vi "DriveModuleControl.vi"(8 "error in":errorcluster, 9 "Actual State":T1={"Speed"=0.0, "Angle"={"VALUE"=0.0, "COS"=1.0, "SIN"=0.0}} {"Angle"."SIN" format="%13.4f"; "Angle"."COS" format="%13.4f"; "Angle"."VALUE" format="%13.4f"}, 10 "Desired State":T1={"Speed"=0.0, "Angle"={"VALUE"=0.0, "COS"=1.0, "SIN"=0.0}} {"Angle"."SIN" format="%13.4f"; "Angle"."COS" format="%13.4f"; "Angle"."VALUE" format="%13.4f"}, 11 "ModualNamePrefix":i32) -> (0 "error out":errorcluster)   [LabVIEW 2023]
uses:
  <vilib>/Rock Robotics/WPI/ThirdParty/JAS_Junk/TrajLib/TypeDef/SWERVE_DRIVE_MODULE_STATE.ctl
  <vilib>/Rock Robotics/WPI/ThirdParty/JAS_Junk/TrajLib/TypeDef/ROTATION2D.ctl
  <vilib>/Rock Robotics/WPI/ThirdParty/JAS_Junk/TrajLib/Rotation2d_Minus.vi
  <vilib>/Rock Robotics/WPI/ThirdParty/JAS_Junk/TrajLib/Rotation2d_GetRadians.vi
  <vilib>/Rock Robotics/WPI/ThirdParty/JAS_Junk/TrajLib/SwerveModuleState_New.vi
  <vilib>/Rock Robotics/WPI/ThirdParty/JAS_Junk/TrajLib/Rotation2d_RotateBy.vi
  <vilib>/Rock Robotics/WPI/ThirdParty/JAS_Junk/TrajLib/Rotation2d_CreateAngle.vi
  <vilib>/Rock Robotics/WPI/ThirdParty/JAS_Junk/TrajLib/SimpleMotorFF_Calculate.vi
  <vilib>/Rock Robotics/WPI/ThirdParty/JAS_Junk/TrajLib/PIDController_AtSetpoint.vi
  <vilib>/Rock Robotics/WPI/ThirdParty/JAS_Junk/TrajLib/PIDController_SetPIDF.vi
  <vilib>/Rock Robotics/WPI/ThirdParty/JAS_Junk/TrajLib/PIDController_SetDerivativeFilter.vi
  <vilib>/Rock Robotics/WPI/ThirdParty/JAS_Junk/TrajLib/PIDController_SetIntegratorRange.vi
  <vilib>/Rock Robotics/WPI/ThirdParty/JAS_Junk/TrajLib/PIDController_SetTolerancePandV.vi
  <vilib>/Rock Robotics/WPI/ThirdParty/JAS_Junk/TrajLib/PIDController_DisableContinousInput.vi
  <vilib>/Rock Robotics/WPI/ThirdParty/JAS_Junk/TrajLib/PIDController_EnableContinousInput.vi
  <vilib>/Rock Robotics/WPI/ThirdParty/JAS_Junk/TrajLib/PIDController_Reset.vi
  <vilib>/Rock Robotics/WPI/ThirdParty/JAS_Junk/TrajLib/PIDController_New.vi
  <vilib>/Rock Robotics/WPI/ThirdParty/JAS_Junk/TrajLib/PIDController_SetOutputLimits.vi
  <vilib>/Rock Robotics/WPI/ThirdParty/JAS_Junk/TrajLib/VI/PIDController_SetIntegratorZone.vi
  <vilib>/Rock Robotics/WPI/ThirdParty/JAS_Junk/TrajLib/SlewRateLimiter_New.vi
  <vilib>/Rock Robotics/WPI/ThirdParty/JAS_Junk/TrajLib/SlewRateLimiter_Reset.vi
  <vilib>/Rock Robotics/WPI/ThirdParty/JAS_Junk/TrajLib/SlewRateLimiter_Calculate.vi
  <vilib>/Rock Robotics/WPI/ThirdParty/JAS_Junk/TrajLib/SlewRateLimiter_SetRate.vi
  <vilib>/Rock Robotics/WPI/ThirdParty/JAS_Junk/TrajLib/Rotation2d_UnaryMinus.vi
  <vilib>/Rock Robotics/WPI/ThirdParty/JAS_Junk/TrajLib/Rotation2d_CreateXY.vi
  <vilib>/Rock Robotics/WPI/ThirdParty/JAS_Junk/TrajLib/PIDController_NewPeriod.vi
  <vilib>/Rock Robotics/WPI/ThirdParty/JAS_Junk/TrajLib/Util_GetTime.vi
  <vilib>/Rock Robotics/WPI/ThirdParty/JAS_Junk/TrajLib/Util_CalcDist.vi
  <vilib>/Rock Robotics/SystemInterfaces/NetworkCommunication/NetComm_UsageReport_report.vi
  <vilib>/Rock Robotics/WPI/ThirdParty/JAS_Junk/TrajLib/VI/Util_GetTime_U32.vi
  DriveGlobal.vi
  <vilib>/Rock Robotics/SystemInterfaces/Utilities/FPGA_UtilitiesRead LocalTime.vi
  <vilib>/Rock Robotics/WPI/ThirdParty/JAS_Junk/TrajLib/VI/Util_GetTime_U64.vi
  <vilib>/Rock Robotics/WPI/ThirdParty/Phoenix6/Phoenix6_Device_RefNumRegistryGet.vi
  <vilib>/Rock Robotics/WPI/MotorControl/WPI_MotorControlRefNum Registry Get.vi
  <vilib>/Rock Robotics/WPI/ThirdParty/JAS_Junk/TrajLib/Globals/Util_LibraryGlobals.vi
  <vilib>/Rock Robotics/WPI/ThirdParty/JAS_Junk/TrajLib/PIDController_AdvCalculate_FF_Sp_Pv.vi
  <vilib>/Rock Robotics/WPI/ThirdParty/JAS_Junk/TrajLib/Trajectory_Library.lvlib
  <vilib>/Rock Robotics/Network Tables/NT Write Number.vi
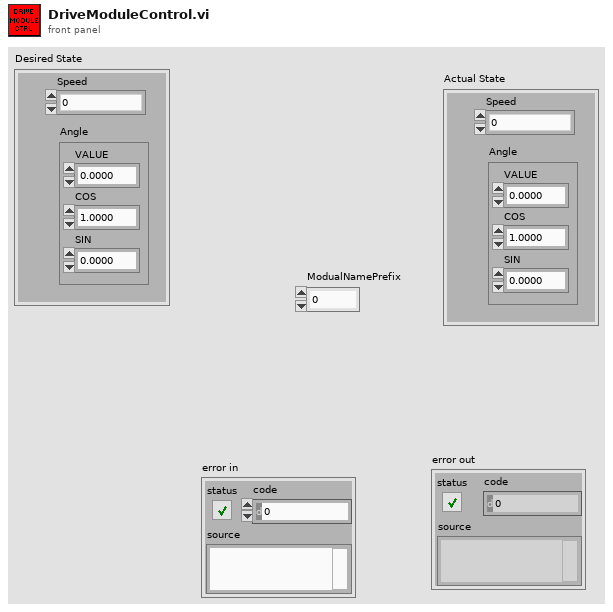
[diagram p1: front panel]
types:
  T1 = typedef "Trajectory_Library.lvlib/SWERVE_DRIVE_MODULE_STATE.ctl" = cluster{"Speed":dbl, "Angle":T2}
  T2 = typedef "Trajectory_Library.lvlib/ROTATION2D.ctl" = cluster{"VALUE":dbl, "COS":dbl, "SIN":dbl}
  T3 = typedef "WPI_MotorControlDeviceRef.ctl" = cluster{"DeviceStatus":errorcluster, "Type":T4, "PWM":cluster{"PWM Channel":T5, "DeadBand":T6}, "CAN":cluster{"Device Number":u8, "SetOutput VI Ref":variant, "GetOutput VI Ref":variant, "Enable VI Ref":variant, "Disable VI Ref":variant, "Data":variant}, "Invert":bool, "DIO PWM":cluster{"PWM \"Enable\" Channel":T5, "DIOChannel":T7, "PWM Rate":dbl}}
  T4 = typedef "WPI_MotorControlType.ctl" = enum16{"PWM", "CAN", "DIO PWM"}
  T5 = typedef "FPGA_DIOPWMChannel.ctl" = enum8{"PWM 0", "PWM 1", "PWM 2", "PWM 3", "PWM 4", "PWM 5", "PWM 6", "PWM 7", "PWM 8", "PWM 9", "PWM MXP 0", "PWM MXP 1", "PWM MXP 2", "PWM MXP 3", "PWM MXP 4", "PWM MXP 5", "PWM MXP 6", "PWM MXP 7", "PWM MXP 8", "PWM MXP 9", "Invalid"}
  T6 = typedef "WPI_PWMDeadband.ctl" = cluster{"Name":string, "maxPositivePwm":i32, "minPositivePwm":i32, "centerPwm":i32, "maxNegativePwm":i32, "minNegativePwm":i32, "angularRange":u16}
  T7 = typedef "FPGA_DIOChannel.ctl" = enum8{"DIO 0", "DIO 1", "DIO 2", "DIO 3", "DIO 4", "DIO 5", "DIO 6", "DIO 7", "DIO 8", "DIO 9", "DIO MXP 0", "DIO MXP 1", "DIO MXP 2", "DIO MXP 3", "DIO MXP 4", "DIO MXP 5", "DIO MXP 6", "DIO MXP 7", "DIO MXP 8", "DIO MXP 9", "DIO MXP 10", "DIO MXP 11", "DIO MXP 12", "DIO MXP 13", "DIO MXP 14", "DIO MXP 15", "SPI Port CS1", "SPI Port CS2", "SPI Port CS3", "SPI Port MISO", "SPI Port MOSI", "Invalid"}
  T8 = typedef "Trajectory_Library.lvlib/SIMPLE_MOTOR_FF.ctl" = cluster{"Ks":dbl, "Kv":dbl, "Ka":dbl, "KnInv":dbl}
  T9 = typedef "Trajectory_Library.lvlib/PID_ADV_LIMITS.ctl" = cluster{"MaxInput":dbl, "MinInput":dbl, "Continuous":bool, "MaxOutput":dbl, "MinOutput":dbl}
  T10 = typedef "Trajectory_Library.lvlib/PID_ADV_TUNING.ctl" = cluster{"Kf":dbl, "Kp":dbl, "Ki":dbl, "Kd":dbl, "MaximumIntegral":dbl, "MinimumIntegral":dbl, "Filter Derivative":bool, "IntegralZone":dbl}
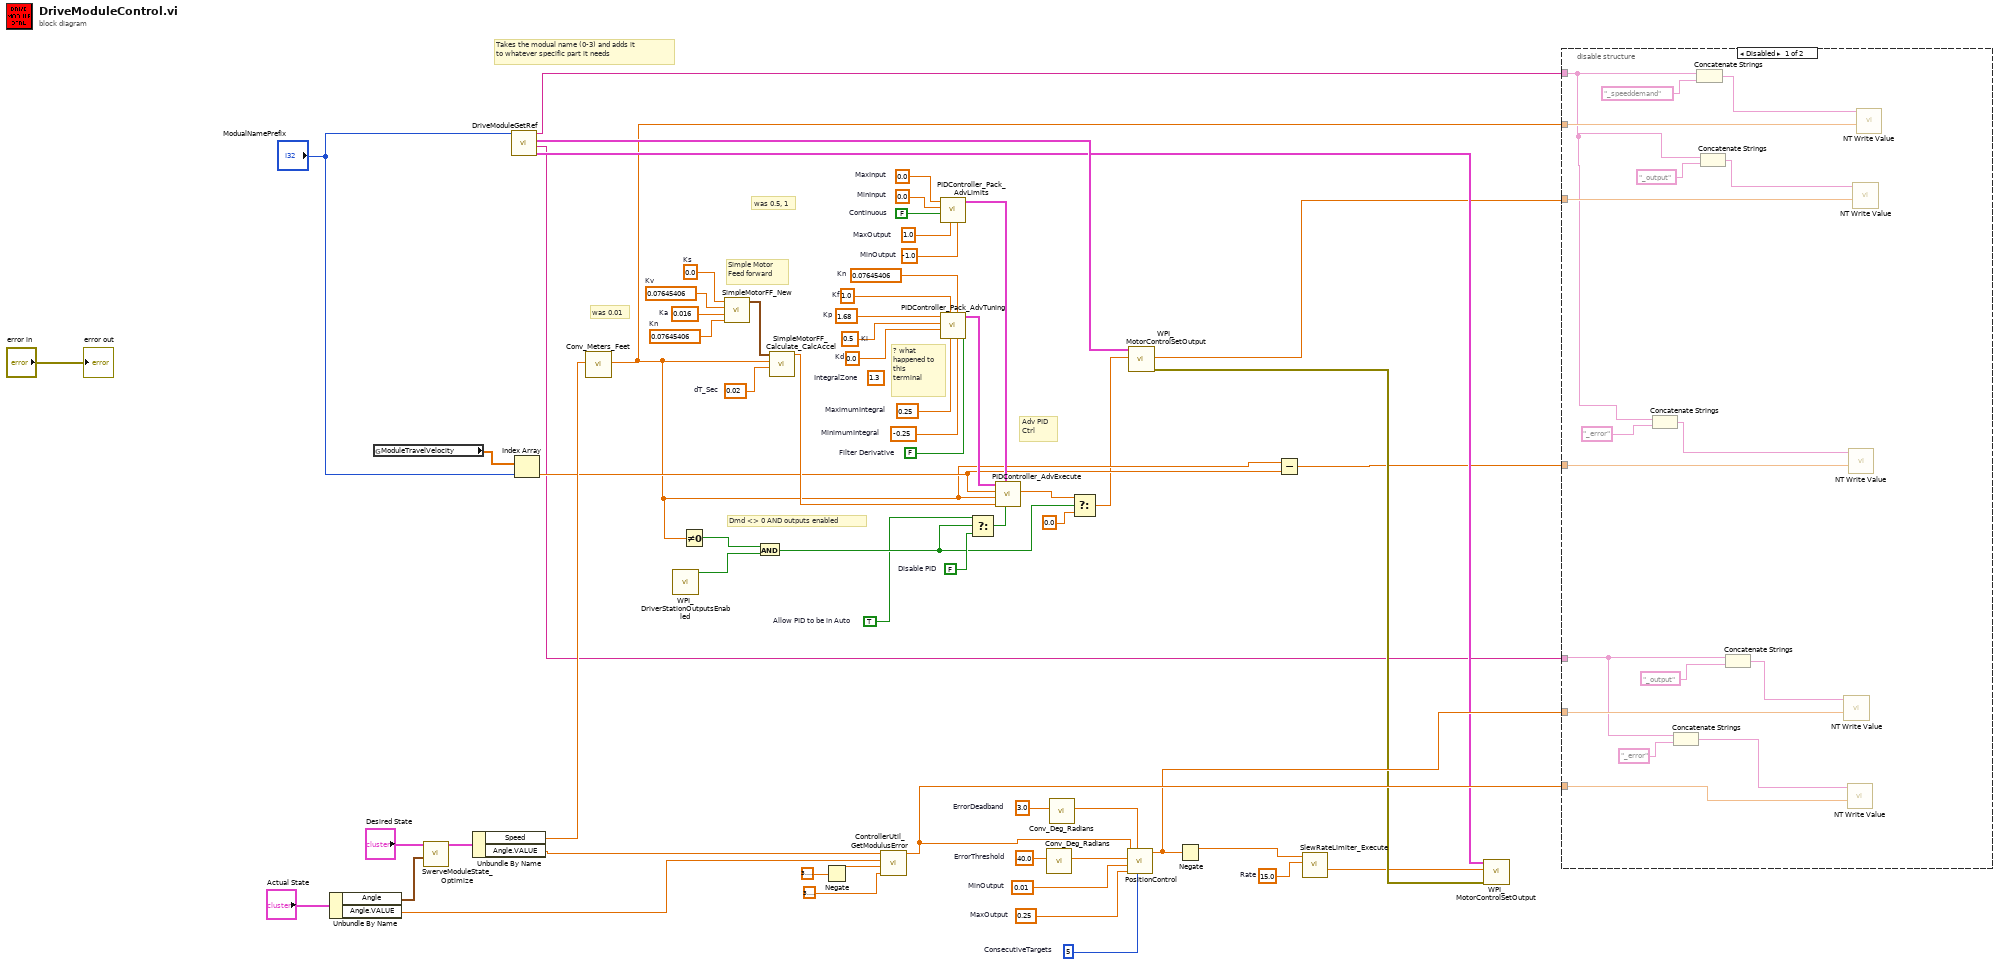
[diagram p0: block diagram]
diagram:
  (unwired) 1.3  # IntegralZone
  w5 = 15.0  # Rate
  w6 = TRUE  # Allow PID to be in Auto
  w8 = FALSE  # Disable PID
  w18 = 0.07645406  # Kn
  w35 = 1.68  # Kp
  w34 = 0.5  # Ki
  w33 = 0.0  # Kd
  w32 = 1.0  # Kf
  w31 = 0.25  # MaximumIntegral
  w30 = -0.25  # MinimumIntegral
  w29 = FALSE  # Filter Derivative
  w27 = 0.0  # MinInput
  w26 = FALSE  # Continuous
  w25 = 1.0  # MaxOutput
  w28 = -1.0  # MinOutput
  w24 = 0.0  # MaxInput
  w44 = 0.07645406  # Kn
  w43 = 0.02  # dT_Sec
  w41 = 0.0  # Ks
  w40 = 0.07645406  # Kv
  w39 = 0.016  # Ka
  w53 = 5  # ConsecutiveTargets
  w51 = 0.25  # MaxOutput
  w54 = 0.01  # MinOutput
  w48 = 40.0  # ErrorThreshold
  w50 = 3.0  # ErrorDeadband
  # "was 0.01"
  # "? what happened to this terminal"
  # "was 0.5, 1"
  # "Dmd <> 0 AND outputs enabled"
  # "Adv PID\nCtrl"
  # "Simple Motor\nFeed forward"
  # "Takes the modual name (0-3) and adds it \nto whatever specific part it needs"
  n1 = Unbundle By Name("Actual State") -> ("Angle"=w61:T2, "Angle.VALUE"=w57:dbl)
  n2 = global read "DriveGlobal.vi" "ModuleTravelVelocity"() -> (w20:dbl[])
  n3 = call <vilib>:"SwerveModuleState_Optimize.vi"("CurrentAngle"=w61, "Desired State"="Desired State") -> ("out SWERVE_DRIVE_MODULE_STATE"=w59:T1)  [unwired: 9 in]
  n4 = Unbundle By Name(w59) -> ("Speed"=w45:dbl, "Angle.VALUE"=w58:dbl)
  n5 = call "DriveModuleGetRef.vi"("ModualNamePrefix"="ModualNamePrefix") -> ("SpinMot"=w36:T3, "SpinStr"=w1:string, "TravMot"=w37:T3, "TravStr"=w2:string)  [unwired: 5 in, 2 out]
  n6 = Index Array(array=w20, index="ModualNamePrefix") -> (element=w17:dbl)
  n7 = call <vilib>:"Conv_Meters_Feet.vi"("Meters"=w45) -> ("Feet"=w15:dbl)  [unwired: 10 in]
  n8 = call <vilib>:"WPI_DriverStationOutputsEnabled.vi"() -> ("OutputsEnabled?"=w11:bool)  [unwired: 10 in, 1 out]
  n9 = Not Equal To 0?(x=w15) -> (x != 0?=w10:bool)
  n10 = call <vilib>:"SimpleMotorFF_New.vi"("Kn"=w44, "Ka"=w39, "Kv"=w40, "Ks"=w41) -> ("SIMPLE_MOTOR_FF"=w42:T8)  [unwired: 7 in]
  n11 = And(x=w10, y=w11) -> (x .and. y?=w7:bool)
  n12 = call <vilib>:"SimpleMotorFF_Calculate_CalcAccel.vi"("dT_Sec"=w43, "VelSp"=w15, "SIMPLE_MOTOR_FF"=w42) -> ("FeedForward"=w21:dbl)  [unwired: 8 in]
  n13 = Negate(x=3.141592653589793) -> (-x=w60:dbl)
  n14 = call <vilib>:"ControllerUtil_GetModulusError.vi"("Maximum_Input"=3.141592653589793, "Minimum_Input"=w60, "Measurerment(PV)"=w57, "Reference(SP)"=w58) -> ("Error"=w52:dbl)  [unwired: 7 in]
  n15 = call <vilib>:"PIDController_Pack_AdvLimits.vi"("MinOutput"=w28, "MaxOutput"=w25, "Continuous"=w26, "MinInput"=w27, "MaxInput"=w24) -> ("Adv PID Limits"=w22:T9)  [unwired: 6 in]
  n16 = call <vilib>:"PIDController_Pack_AdvTuning.vi"("Filter Derivative"=w29, "MinimumIntegral"=w30, "Kn"=w18, "MaximumIntegral"=w31, "Kf"=w32, "Kd"=w33, "Ki"=w34, "Kp"=w35) -> ("Adv PID Tuning"=w23:T10)  [unwired: 3 in]
  n17 = Select(t=w6, s=w7, f=w8) -> (s? t:f=w9:bool)
  n18 = call <vilib>:"PIDController_AdvExecute.vi"("Auto"=w9, "Adv PID Limits"=w22, "FF-FeedForward"=w21, "SP-SetPoint"=w15, "PV-Measurement"=w17, "Adv PID Tuning"=w23) -> ("CO-ControlOutput"=w13:dbl)  [unwired: 3 in, 2 out]
  n19 = call <vilib>:"Conv_Deg_Radians.vi"("Degress"=w48) -> ("Radians"=w47:dbl)  [unwired: 10 in]
  n20 = call <vilib>:"Conv_Deg_Radians.vi"("Degress"=w50) -> ("Radians"=w49:dbl)  [unwired: 10 in]
  n21 = Select(t=w13, s=w7, f=0.0 ("t")) -> (s? t:f=w14:dbl)
  n22 = call "PositionControl.vi"("ConsecutiveTargets"=w53, "ErrorDeadband"=w49, "MaxOutput"=w51, "MinOutput"=w54, "ErrorThreshold"=w47, "Error"=w52) -> ("OutputValue"=w46:dbl)  [unwired: 3 in, 2 out]
  n23 = call <vilib>:"WPI_MotorControlSetOutput.vi"("Output"=w14, "MotorControlDevRef"=w37) -> ("error out"=w38:errorcluster)  [unwired: 7 in, 2 out]
  n24 = Negate(x=w46) -> (-x=w4:dbl)
  n25 = Subtract(x=w15, y=w17) -> (x-y=w16:dbl)
  n26 = call <vilib>:"SlewRateLimiter_Execute.vi"("PositiveRate"=w5, "Input"=w4) -> ("Output"=w3:dbl)  [unwired: 8 in, 1 out]
  n27 = call <vilib>:"WPI_MotorControlSetOutput.vi"("error in (no error)"=w38, "Output"=w3, "MotorControlDevRef"=w36) -> ()  [unwired: 6 in, 3 out]
  n28 = disable-structure shown="Disabled" {
    disable-tunnel: w52 -> [w81 _]
    disable-tunnel: w46 -> [w80 _]
    disable-tunnel: w16 -> [w79 _]
    disable-tunnel: w15 -> [w78 _]
    disable-tunnel: w14 -> [w77 _]
    disable-tunnel: w2 -> [w70 _]
    disable-tunnel: w1 -> [w65 _]
    frame Disabled {
      n29 = Concatenate Strings(w70, "_error" ("refnum name")) -> (w71:string)
      n30 = Concatenate Strings(w65, "_error" ("refnum name")) -> (w66:string)
      n31 = Concatenate Strings(w70, "_speeddemand" ("refnum name")) -> (w75:string)
      n32 = Concatenate Strings(w70, "_output" ("refnum name")) -> (w73:string)
      n33 = Concatenate Strings(w65, "_output" ("refnum name")) -> (w68:string)
      n34 = call-poly <vilib>:"NT Write Value.vi"("value"=w80, "name"=w68) -> ()  [unwired: 9 in, 1 out]
      n35 = call-poly <vilib>:"NT Write Value.vi"("value"=w81, "name"=w66) -> ()  [unwired: 9 in, 1 out]
      n36 = call-poly <vilib>:"NT Write Value.vi"("value"=w79, "name"=w71) -> ()  [unwired: 9 in, 1 out]
      n37 = call-poly <vilib>:"NT Write Value.vi"("value"=w77, "name"=w73) -> ()  [unwired: 9 in, 1 out]
      n38 = call-poly <vilib>:"NT Write Value.vi"("value"=w78, "name"=w75) -> ()  [unwired: 9 in, 1 out]
    }
    frame Enabled {
    }
  }
  "error out" <- "error in"
